vi "Construct.vi"(0 "Component Config File":path) -> (4 "Component":refnum<class "Component.lvclass">)   [LabVIEW 2017, in "CL_G3_VIComponentBuilder.lvlib" / "Component.lvclass"]
doc: "Brings the Component object into existence and sets the initial values according to the Component Config File."
uses:
  Component.lvclass
  Component.lvclass/Component.ctl
  Accessors/Write Component Config File.vi
  Accessors/Write Component Operations Errors.vi
  Accessors/Write Component Path.vi
  <vilib>/Utility/config.llb/NI_LVConfig.lvlib
  CL_G3_VIComponentBuilder.lvlib
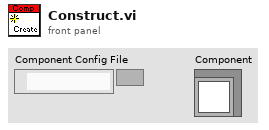
[diagram p1: front panel]
types:
  T1 = typedef "NI_LVConfig.lvlib/Config Data RefNum.ctl" = refnum<k1>
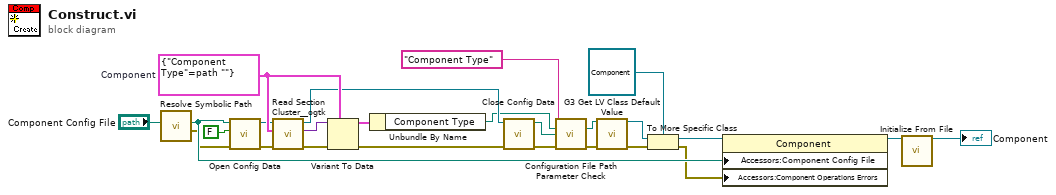
[diagram p0: block diagram]
diagram:
  w23 = cluster{"Component Type":path} {"Component Type"=path ""}  # Component
  n1 = call "Resolve Symbolic Path.vi"("Path In"="Component Config File") -> ("error out"=w1:errorcluster, "Path Out"=w4:path)  [unwired: 9 in]
  n2 = call <vilib>:"Open Config Data.vi"("error in (no error)"=w1, "create file if necessary (T)"=FALSE, "configuration file path"=w4) -> ("error out"=w17:errorcluster, "refnum"=w21:T1)  [unwired: 6 in, 1 out]
  n3 = call <userlib>:"Read Section Cluster__ogtk.vi"("error in (no error)"=w17, "Section Formatted Cluster Type"=w23, "refnum"=w21) -> ("error out"=w19:errorcluster, "Section Formatted Cluster"=w24:variant, "dup refnum"=w20:T1)  [unwired: 4 in, 2 out]
  n4 = Variant To Data(error in=w19, type=w23, Variant=w24) -> (data=w22:cluster{"Component Type":path}, error out=w18:errorcluster)
  n5 = Unbundle By Name(w22) -> ("Component Type"=w10:path)
  n6 = call <vilib>:"Close Config Data.vi"("error in (no error)"=w18, "refnum"=w20) -> ("error out"=w7:errorcluster, "file path"=w9:path)  [unwired: 8 in]
  n7 = call "Configuration File Path Parameter Check.vi"("Parameter Name"="Component Type", "Specified Path in Configuration File"=w10, "Configuration File Path"=w9, "error in (no error)"=w7) -> ("dup Specified Path in Configuration File"=w8:path, "error out"=w6:errorcluster)  [unwired: 9 in, 1 out]
  n8 = call "G3 Get LV Class Default Value.vi"("Export Type"=w8, "error in (no error)"=w6) -> ("LabVIEW Object out"=w16:refnum<class>, "error out"=w15:errorcluster)  [unwired: 12 in]
  n9 = To More Specific Class(target class=refnum<class "Component.lvclass"> refnum ("Component"), reference=w16, error in=w15) -> (specific class reference=w13:refnum<class "Component.lvclass">, error out=w3:errorcluster)
  n10 = property class="Component"(reference=w13, "Accessors:Component Config File"=w4, "Accessors:Component Operations Errors"=w3) -> (reference out=w2:refnum<class "Component.lvclass">)  [unwired: 1 in, 1 out]
  n11 = call-dynamic "Initialize From File.vi"("Component in"=w2) -> ("Component out"=→"Component":refnum<class "Component.lvclass">)  [unwired: 14 in]
